vi "换刀.vi"(8 "error in (no error)":errorcluster caption="错误输入（无错误）", 11 "加工类（抽象） 输入":refnum<class "加工类（抽象）.lvclass"> caption="DNL_LabVIEW Object in") -> (0 "error out":errorcluster caption="错误输出", 3 "加工类（抽象） 输出":refnum<class "加工类（抽象）.lvclass"> caption="DNL_LabVIEW Object out")   [LabVIEW 2011, in "加工类（抽象）.lvclass"]
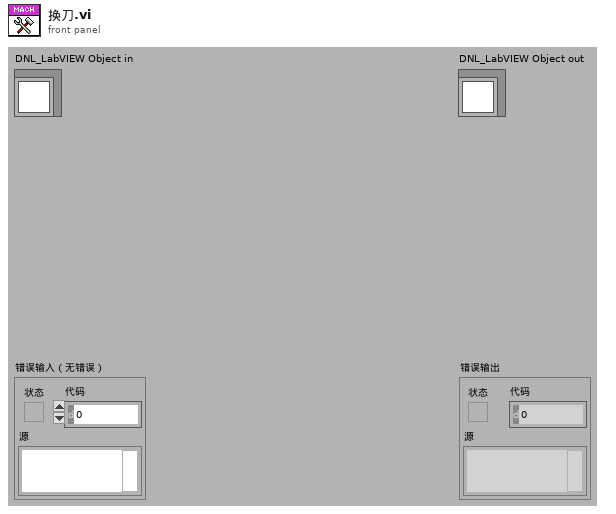
[diagram p1: front panel]
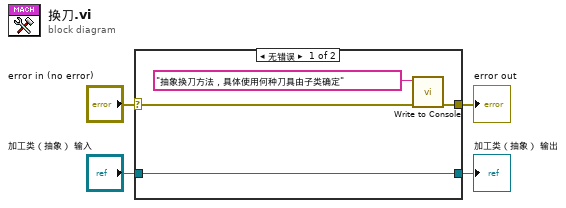
[diagram p0: block diagram]
diagram:
  n1 = case shown="无错误" "error in (no error)" {
    selector: "error in (no error)" -> [w7 w10]
    tunnel: [w6 w10] -> w3
    tunnel: [w8 w9] -> w1
    tunnel: "加工类（抽象） 输入" -> [w8 w9]
    frame No Error {
      n2 = call "Write to Console.vi"("error in (no error)"=w7, "Input"="抽象换刀方法，具体使用何种刀具由子类确定") -> ("error out"=w6:errorcluster)  [unwired: 9 in]
    }
    frame Error {
    }
  }
  "error out" <- w3
  "加工类（抽象） 输出" <- w1
